vi "qpsk.vi"() -> ()   [LabVIEW 2014]
panel:
  out "Waveform Graph":dynamicdata(graph)
  out "0, 2":i16
  out "0, 1":i16
  out "number":u32
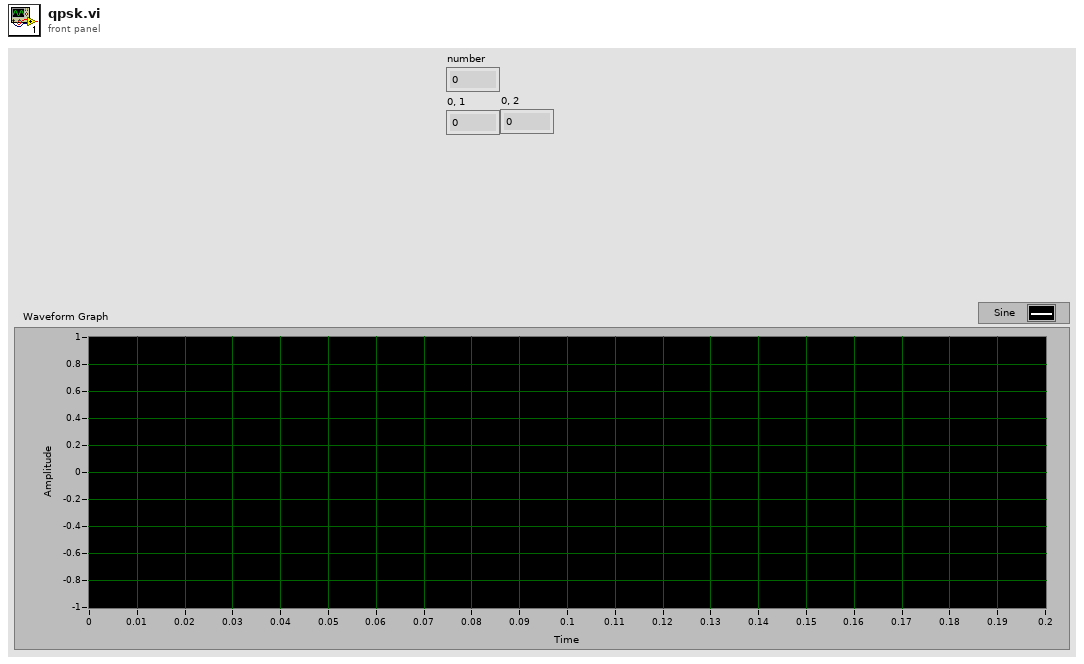
[diagram p1: front panel]
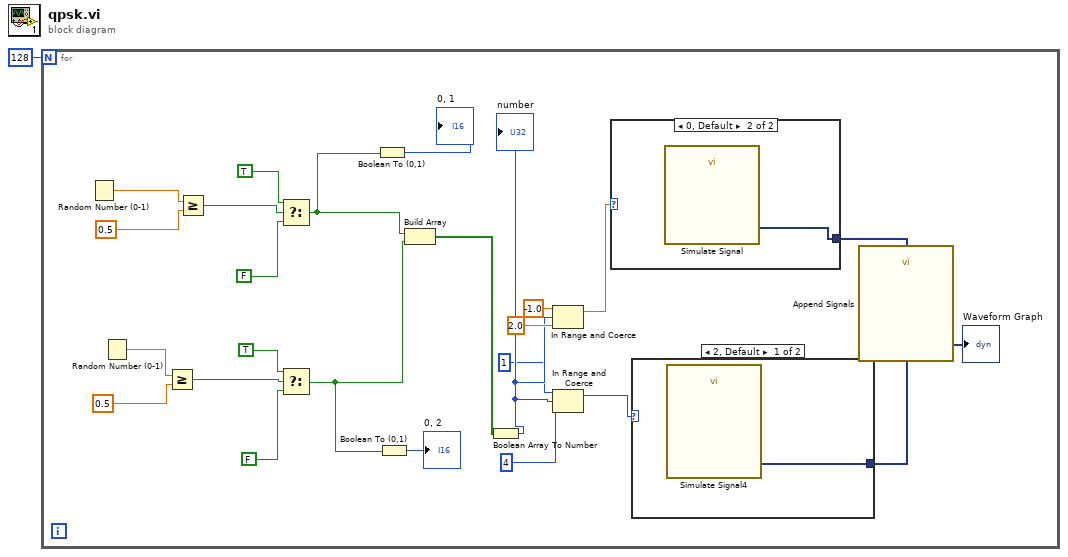
[diagram p0: block diagram]
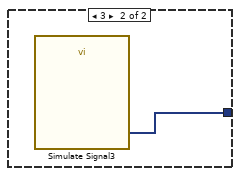
[diagram p2: hidden frame]
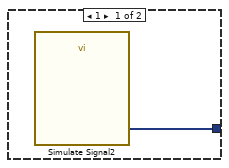
[diagram p3: hidden frame]
diagram:
  n1 = for {
    N: 128 -> [_]
    n2 = Random Number (0-1)() -> (number: 0 to 1=w24:dbl)
    n3 = Random Number (0-1)() -> (number: 0 to 1=w26:dbl)
    n4 = Greater Or Equal?(x=w26, y=0.5) -> (x >= y?=w21:bool)
    n5 = Greater Or Equal?(x=w24, y=0.5) -> (x >= y?=w22:bool)
    n6 = Select(t=TRUE, s=w22, f=FALSE) -> (s? t:f=w16:bool)
    n7 = Select(t=TRUE, s=w21, f=FALSE) -> (s? t:f=w14:bool)
    n8 = Boolean To (0,1)(Boolean=w16) -> (0, 1=→"0, 1":i16)
    n9 = Boolean To (0,1)(Boolean=w14) -> (0, 1=→"0, 2":i16)
    n10 = Build Array(w16, w14) -> (w12:bool[])
    n11 = Boolean Array To Number(Boolean array=w12) -> (number=w6:u32)
    "number" <- w6
    n12 = In Range and Coerce(upper limit=-1.0, x=w6, lower limit=2.0) -> (coerced(x)=w3:dbl)  [unwired: 1 out]
    n13 = In Range and Coerce(upper limit=u32 1, x=w6, lower limit=u32 4) -> (coerced(x)=w2:u32)  [unwired: 1 out]
    n14 = case shown="0, Default" w3 {
      tunnel: [w29 w30] -> w11
      frame 1 {
        n15 = call "Simulate Signal2"() -> ("Sine"=w29:dynamicdata)  [unwired: 14 in, 1 out]
      }
      frame 0, Default {
        n16 = call "Simulate Signal"() -> ("Sine"=w30:dynamicdata)  [unwired: 14 in, 1 out]
      }
    }
    n17 = case shown="2, Default" w2 {
      tunnel: [w27 w28] -> w10
      frame 2, Default {
        n18 = call "Simulate Signal4"() -> ("Sine"=w27:dynamicdata)  [unwired: 14 in, 1 out]
      }
      frame 3 {
        n19 = call "Simulate Signal3"() -> ("Sine"=w28:dynamicdata)  [unwired: 14 in, 1 out]
      }
    }
    n20 = call "Append Signals"("Input Signal B"=w10, "Input Signal A"=w11) -> ("Appended Signals"=→"Waveform Graph":dynamicdata)  [unwired: 8 in, 1 out]
  }
